vi "通信模块_串口调试工具.vi"() -> ()   [LabVIEW 2015]
uses:
  <vilib>/Instr/_visa.llb/VISA Find Search Mode.ctl
  <vilib>/event_ctls.llb/eventvkey.ctl
  <vilib>/Instr/_visa.llb/VISA Configure Serial Port (Instr).vi
panel:
  in  "1A":bool caption="进制"
  in  "2 3":string
  in  "2 2":bool
  in  "1 3":string
  in  "1 2":bool
  in  "5 3":bool
  in  "4 3":bool
  in  "3 3":bool
  in  "5 2":string
  in  "4 2":string
  in  "3 2":string
  in  "ATI":bool
  in  "CGMM":bool
  in  "CGMI":bool
  in  "ATE1":bool
  in  "批量AT":bool
  in  "保存":bool
  in  "时间显示":bool caption="进制"
  in  "CGMR":bool
  in  "回车":bool=TRUE caption="进制"
  in  "十六进制":bool caption="进制"
  in  "2":string
  in  "2":bool
  in  "1":string
  in  "1":bool
  in  "语音":bool
  in  "短信":bool
  in  "ATE0":bool
  in  "CIMI":bool
  in  "CREG":bool
  in  "CPIN?":bool
  in  "CSQ":bool
  in  "5":bool
  in  "4":bool
  in  "3":bool
  in  "AT+？ 5":bool
  in  "5":string
  in  "4":string
  in  "3":string
  in  "AT+? 5":string
  in  "手动发送":bool
  in  "周期":u16=100
  in  "自动发送":bool
  in  "发送区":string
  in  "AT+? 4":bool
  in  "AT+? 4":string
  out "发送":string
  in  "窗口":string
  in  "AT+？ 3":bool
  in  "AT+? 3":string
  in  "AT+？ 2":bool
  in  "AT+? 2":string
  in  "AT+？":bool
  in  "AT+? 1":string
  in  "AT":bool
  in  "清空":bool
  out "VISA":refnum<visa-resource-name>
  in  "端口":string(combo)="COM2"
  in  "波特率":string(combo)="115200"
  out "布尔":bool
  in  "串口开关":bool
  # "毫秒"
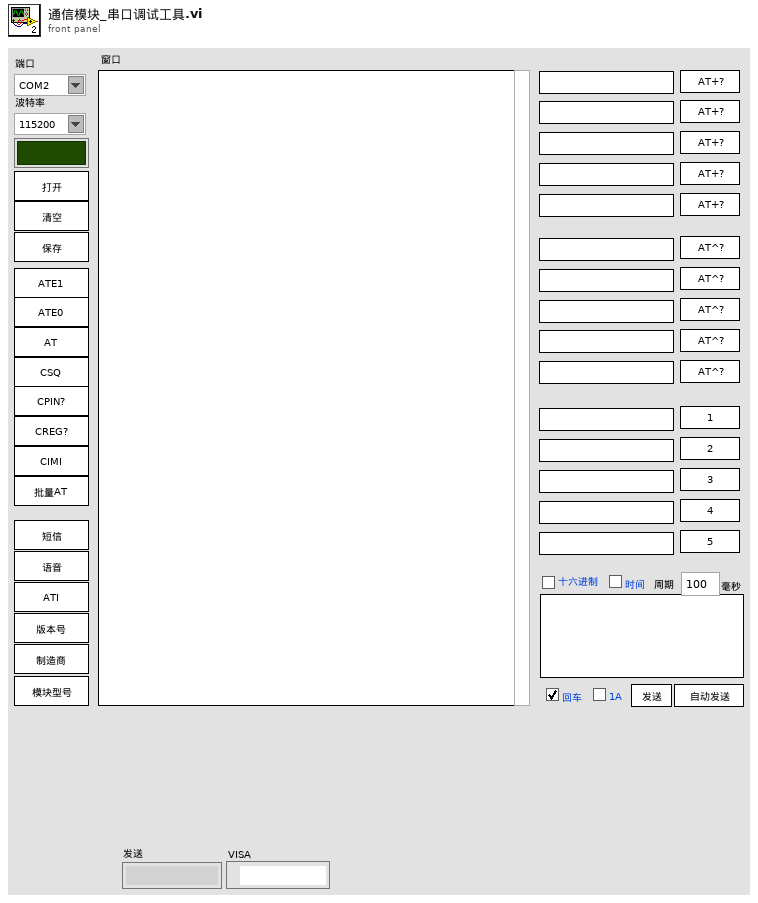
[diagram p1: front panel]
types:
  T1 = typedef "VISA Find Search Mode.ctl" = u32
  T2 = typedef "eventvkey.ctl" = enum16{"ASCII", "Enter", "Return", "Shift", "Ctrl", "Alt", "Cmd", "Opt", "Caps", "NumLock", "Clear", "Break", "Up", "Down", "Left", "Right", "Insert", "Delete", "Home", "End", "PageUp", "PageDown", "Escape", "Help", "Pause", "ScrollLock", "F1", "F2", "F3", "F4", "F5", "F6", "F7", "F8", "F9", "F10", "F11", "F12", "F13", "F14", "F15", "F16", "F17", "F18", "F19", "F20", "F21", "F22", "F23", "F24", "Play", "VolumeUp", "VolumeDown", "Mute", "Two Byte Char"}
  T3 = cluster{"Shift":bool, "Ctrl":bool, "Alt":bool, "Cmd":bool, "Opt":bool}
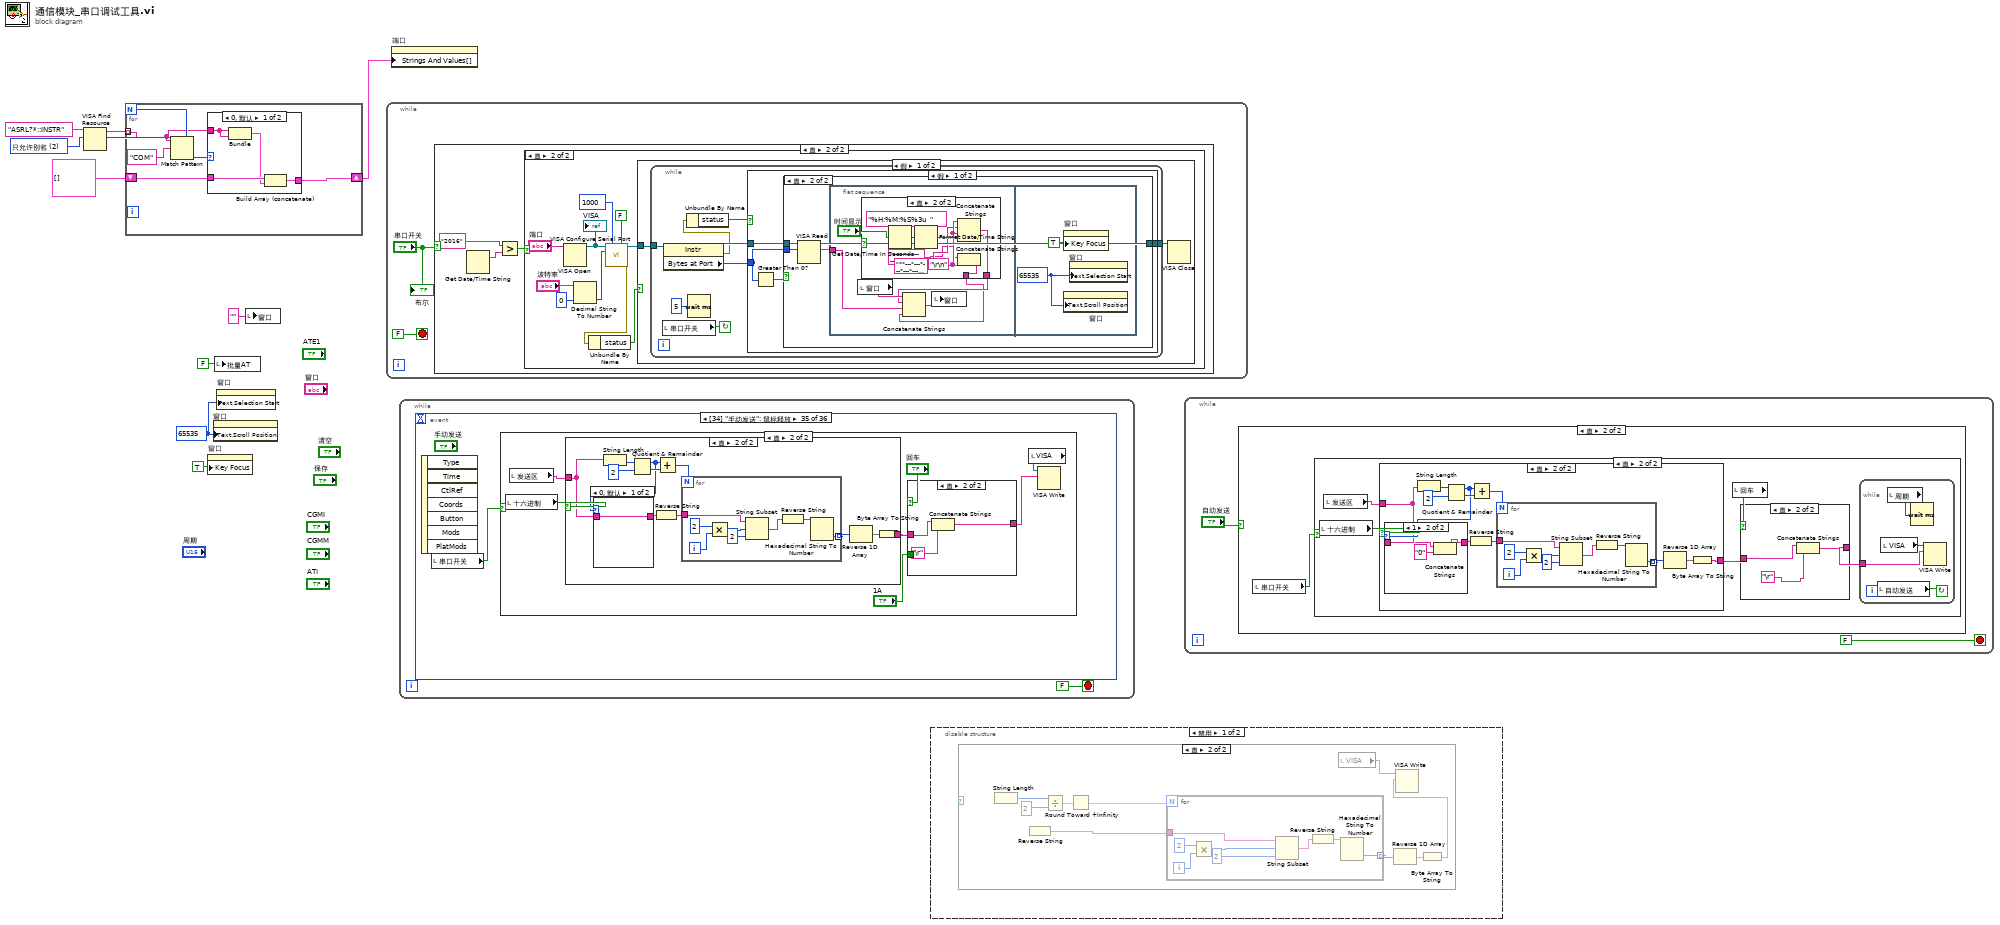
[diagram p0: block diagram]
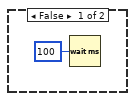
[diagram p3: hidden frame]
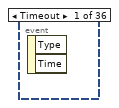
[diagram p10: hidden frame]
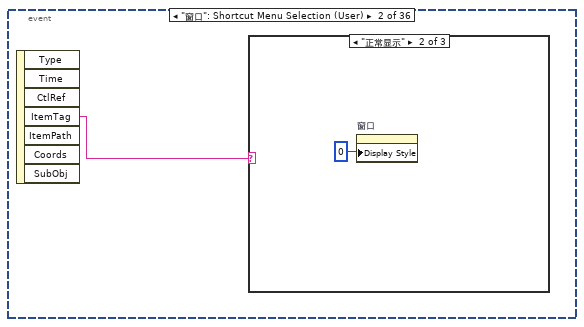
[diagram p11: hidden frame]
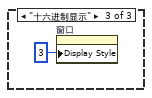
[diagram p13: hidden frame]
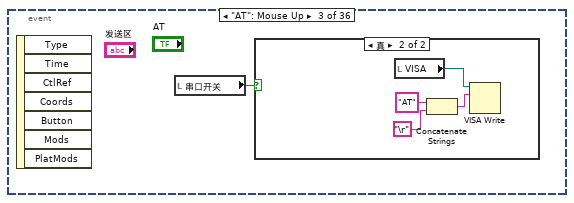
[diagram p14: hidden frame]
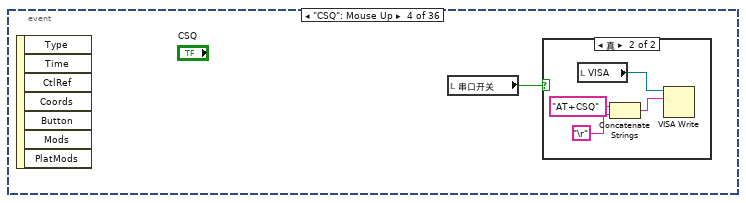
[diagram p16: hidden frame]
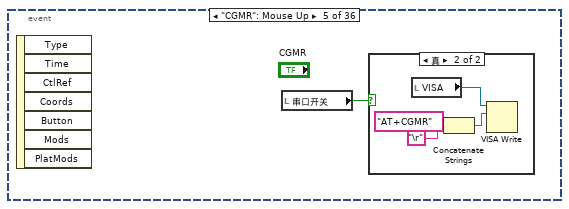
[diagram p18: hidden frame]
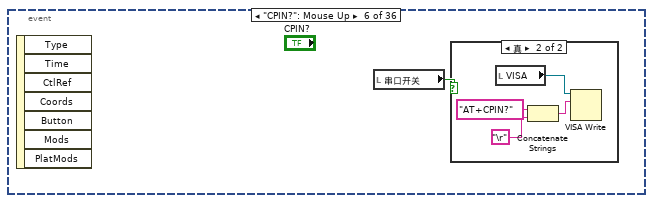
[diagram p20: hidden frame]
diagram:
  w3 = T1 2 items=["仅允许规范名称"=0, "只允许别名"=2, "包含匹配别名"=3, "包含所有别名"=4] ("Search Mode")
  w9 = u32 65535 ("文本.滚动条位置")
  n1 = VISA Find Resource(10:w3, 11:"ASRL?*::INSTR") -> (2:w7:u32, 3:w6:string[])  [unwired: 1 in, 1 out]
  n2 = for {
    N: w7 -> [_]
    tunnel: w6 -> [w13] mode=indexing
    shift-right: [w12] -> w1
    shift-left: cluster{string, string}[] [] -> [w11]
    n3 = Match Pattern(string=w13, regular expression="COM" ("正则表达式")) -> (offset past match=w14:i32)  [unwired: 1 in, 3 out]
    n4 = case shown="0, 默认" w14 {
      tunnel: w11 -> [w19 w20]
      tunnel: w13 -> [w17 _]
      tunnel: [w18 w20] -> w12
      frame 0, Default {
        n5 = Bundle(w17, w17) -> (w16:cluster{string, string})  [unwired: 1 in]
        n6 = Build Array (concatenate)(w19, w16) -> (w18:cluster{string, string}[])
      }
      frame -1 {
      }
    }
  }
  n7 = property on="窗口" class="Str"("Key Focus"=TRUE ("键选中")) -> ()  [unwired: 2 in, 2 out]
  n8 = property on="窗口" class="Str"("Text.Scroll Position"=w9) -> ()  [unwired: 2 in, 2 out]
  n9 = local write "批量AT"(FALSE ("批量AT")) -> ()
  n10 = property on="窗口" class="Str"("Text.Selection Start"=w9) -> ()  [unwired: 2 in, 2 out]
  n11 = local write "窗口"("" ("窗口")) -> ()
  n12 = while {
    stop <- FALSE stop-if-true
    n13 = case shown="真" "串口开关" {
      frame False {
        n14 = Wait (ms)(milliseconds to wait=u32 100 ("等待时间（毫秒）")) -> ()  [unwired: 1 out]
      }
      frame True {
        n15 = Get Date/Time String() -> (date string=w26:string)  [unwired: 3 in, 1 out]
        n16 = Greater?(x="2016", y=w26) -> (0:w24:bool)
        n17 = case shown="真" w24 {
          frame False {
            n18 = Wait (ms)(milliseconds to wait=u32 100 ("等待时间（毫秒）")) -> ()  [unwired: 1 out]
          }
          frame True {
            n19 = VISA Open(VISA resource name="端口") -> (VISA resource name=w37:refnum<visa-resource-name>)  [unwired: 4 in, 1 out]
            "VISA" <- w37
            n20 = Decimal String To Number(string="波特率", default (0L)=u32 0 ("默认(0 I32)")) -> (number=w30:u32)  [unwired: 1 in, 1 out]
            n21 = call-poly "VISA Configure Serial Port"("VISA resource name"=w37, "timeout (10sec)"=u32 1000, "Enable Termination\nChar (T)"=FALSE ("Enable Termination\nChar (T)"), "baud rate (9600)"=w30) -> ("VISA resource name out"=w34:refnum<visa-resource-name>, "error out"=w33:errorcluster)  [unwired: 10 in]
            n22 = Unbundle By Name(w33) -> ("status"=w32:bool)
            n23 = case shown="假" w32 {
              tunnel: w34 -> [w38 _]
              frame False {
                n24 = while {
                  tunnel: [w45] -> w39
                  tunnel: w38 -> [w43]
                  stop <- w47 continue-if-true
                  n25 = local read "串口开关"() -> (w47:bool)
                  n26 = property class="Instr"(reference=w43) -> (reference out=w46:refnum<visa-resource-name>, error out=w41:errorcluster, "Bytes at Port"=w42:u32)  [unwired: 1 in]
                  n27 = Unbundle By Name(w41) -> ("status"=w40:bool)
                  n28 = Wait (ms)(milliseconds to wait=u32 5 ("等待时间（毫秒）")) -> ()  [unwired: 1 out]
                  n29 = case shown="假" w40 {
                    tunnel: w46 -> [w51 w74]
                    tunnel: [w50 w74] -> w45
                    tunnel: w42 -> [w48 _]
                    frame False {
                      n30 = Greater Than 0?(x=w48) -> (x > 0?=w49:bool)
                      n31 = case shown="真" w49 {
                        tunnel: w51 -> [w52 w56]
                        tunnel: w48 -> [_ w55]
                        tunnel: [w52 w54] -> w50
                        frame False {
                        }
                        frame True {
                          n32 = VISA Read(VISA resource name=w56, byte count=w55) -> (VISA resource name out=w54:refnum<visa-resource-name>, read buffer=w53:string)  [unwired: 1 in, 2 out]
                          n33 = flat-sequence {
                            tunnel: w53 -> [w59]
                            frame #0 {
                              n34 = local read "窗口"() -> (w61:string)
                              n35 = case shown="真" "时间显示" {
                                tunnel: [w63 w68] -> w58
                                tunnel: [w63 w66] -> w57
                                frame False {
                                w63 = "" ("date/time string")
                                }
                                frame True {
                                w67 = "\r\n"
                                n36 = Get Date/Time In Seconds() -> (seconds since 1Jan1904=w71:timestamp)
                                n37 = Format Date/Time String(time format string (%c)="%H:%M:%S%3u  " ("时间格式字符串(%c)"), seconds (now)=w71) -> (date/time string=w69:string)  [unwired: 1 in]
                                n38 = Concatenate Strings(w67, "**---*---*---*---*---*---*---*---*---*---*---*---*---*---*---**" ("窗口"), w67, w69) -> (w68:string)
                                n39 = Concatenate Strings("----------------------------------------------------------------" ("窗口"), w67) -> (w66:string)
                                }
                              }
                              n40 = Concatenate Strings(w61, w58, w59, w57) -> (w62:string)
                              n41 = local write "窗口"(w62) -> ()
                            }
                            frame #1 {
                              w72 = u32 65535 ("文本.选择区域:起始")
                              n42 = property on="窗口" class="Str"("Key Focus"=TRUE ("键选中")) -> ()  [unwired: 2 in, 2 out]
                              n43 = property on="窗口" class="Str"("Text.Scroll Position"=w72) -> ()  [unwired: 2 in, 2 out]
                              n44 = property on="窗口" class="Str"("Text.Selection Start"=w72) -> ()  [unwired: 2 in, 2 out]
                            }
                          }
                        }
                      }
                    }
                    frame True {
                    }
                  }
                }
                n45 = VISA Close(VISA resource name=w39) -> ()  [unwired: 1 in, 1 out]
              }
              frame True {
                n46 = flat-sequence {
                  frame #0 {
                    n47 = local read "端口"() -> (w77:string)
                    n48 = Concatenate Strings(w77, "打开失败！" ("字符串")) -> (w75:string)
                    n49 = One Button Dialog(message=w75) -> ()  [unwired: 1 in, 1 out]
                  }
                  frame #1 {
                    n50 = local write "串口开关"(FALSE ("串口开关")) -> ()
                  }
                }
              }
            }
          }
        }
      }
    }
    "布尔" <- "串口开关"
  }
  n51 = property on="端口" class="CmbBox"("Strings And Values[]"=w1) -> ()  [unwired: 2 in, 2 out]
  n52 = while {
    stop <- FALSE stop-if-true
    n53 = event shown="[34] \"手动发送\": 鼠标释放" {
      selector: _ -> [_ _ _ _ _ _ _ _ _ _ _ _ _ _ _ _ _ _ _ _ _ _ _ _ _ _ _ _ _ _ _ _ _ _ _ _]
      dyn-events: _ -> [_ _ _ _ _ _ _ _ _ _ _ _ _ _ _ _ _ _ _ _ _ _ _ _ _ _ _ _ _ _ _ _ _ _ _ _]
      timeout: _ -> [_ _ _ _ _ _ _ _ _ _ _ _ _ _ _ _ _ _ _ _ _ _ _ _ _ _ _ _ _ _ _ _ _ _ _ _]
      event Timeout {
        n54 = event-data() -> ()  [unwired: 1 in, 2 out]
      }
      event "窗口": Shortcut Menu Selection (User) {
        n55 = event-data() -> ("ItemTag"=w80:string)  [unwired: 1 in, 6 out]
        n56 = case shown="\"正常显示\"" w80 {
          frame "假", Default {
          }
          frame "正常显示" {
            n57 = property on="窗口" class="Str"("Display Style"=u32 0 ("显示样式")) -> ()  [unwired: 2 in, 2 out]
          }
          frame "十六进制显示" {
            n58 = property on="窗口" class="Str"("Display Style"=u32 3 ("显示样式")) -> ()  [unwired: 2 in, 2 out]
          }
        }
      }
      event "AT": Mouse Up {
        n59 = event-data() -> ()  [unwired: 1 in, 7 out]
        n60 = local read "串口开关"() -> (w83:bool)
        n61 = case shown="真" w83 {
          frame False {
          }
          frame True {
            n62 = local read "VISA"() -> (w87:refnum<visa-resource-name>)
            n63 = Concatenate Strings("AT" ("字符串"), "\r") -> (w86:string)
            n64 = VISA Write(VISA resource name=w87, write buffer=w86) -> ()  [unwired: 1 in, 3 out]
          }
        }
      }
      event "CSQ": Mouse Up {
        n65 = event-data() -> ()  [unwired: 1 in, 7 out]
        n66 = local read "串口开关"() -> (w88:bool)
        n67 = case shown="真" w88 {
          frame False {
          }
          frame True {
            n68 = local read "VISA"() -> (w92:refnum<visa-resource-name>)
            n69 = Concatenate Strings("AT+CSQ" ("字符串"), "\r") -> (w91:string)
            n70 = VISA Write(VISA resource name=w92, write buffer=w91) -> ()  [unwired: 1 in, 3 out]
          }
        }
      }
      event "CGMR": Mouse Up {
        n71 = event-data() -> ()  [unwired: 1 in, 7 out]
        n72 = local read "串口开关"() -> (w93:bool)
        n73 = case shown="真" w93 {
          frame False {
          }
          frame True {
            n74 = local read "VISA"() -> (w97:refnum<visa-resource-name>)
            n75 = Concatenate Strings("AT+CGMR" ("字符串"), "\r") -> (w96:string)
            n76 = VISA Write(VISA resource name=w97, write buffer=w96) -> ()  [unwired: 1 in, 3 out]
          }
        }
      }
      event "CPIN?": Mouse Up {
        n77 = event-data() -> ()  [unwired: 1 in, 7 out]
        n78 = local read "串口开关"() -> (w98:bool)
        n79 = case shown="真" w98 {
          frame False {
          }
          frame True {
            n80 = local read "VISA"() -> (w102:refnum<visa-resource-name>)
            n81 = Concatenate Strings("AT+CPIN?" ("字符串"), "\r") -> (w101:string)
            n82 = VISA Write(VISA resource name=w102, write buffer=w101) -> ()  [unwired: 1 in, 3 out]
          }
        }
      }
      event "CREG": Mouse Up {
        n83 = event-data() -> ()  [unwired: 1 in, 7 out]
        n84 = local read "串口开关"() -> (w103:bool)
        n85 = case shown="真" w103 {
          frame False {
          }
          frame True {
            n86 = local read "VISA"() -> (w107:refnum<visa-resource-name>)
            n87 = Concatenate Strings("AT+CREG?" ("字符串"), "\r") -> (w106:string)
            n88 = VISA Write(VISA resource name=w107, write buffer=w106) -> ()  [unwired: 1 in, 3 out]
          }
        }
      }
      event "CIMI": Mouse Up {
        n89 = event-data() -> ()  [unwired: 1 in, 7 out]
        n90 = local read "串口开关"() -> (w108:bool)
        n91 = case shown="真" w108 {
          frame False {
          }
          frame True {
            n92 = local read "VISA"() -> (w112:refnum<visa-resource-name>)
            n93 = Concatenate Strings("AT+CIMI" ("字符串"), "\r") -> (w111:string)
            n94 = VISA Write(VISA resource name=w112, write buffer=w111) -> ()  [unwired: 1 in, 3 out]
          }
        }
      }
      event "ATE0": Mouse Up {
        n95 = event-data() -> ()  [unwired: 1 in, 7 out]
        n96 = local read "串口开关"() -> (w113:bool)
        n97 = case shown="真" w113 {
          frame False {
          }
          frame True {
            n98 = local read "VISA"() -> (w117:refnum<visa-resource-name>)
            n99 = Concatenate Strings("ATE0" ("字符串"), "\r") -> (w116:string)
            n100 = VISA Write(VISA resource name=w117, write buffer=w116) -> ()  [unwired: 1 in, 3 out]
          }
        }
      }
      event "短信": Mouse Up {
        n101 = event-data() -> ()  [unwired: 1 in, 7 out]
        n102 = flat-sequence {
          frame #0 {
            n103 = local read "VISA"() -> (w121:refnum<visa-resource-name>)
            n104 = Concatenate Strings("AT+CMGS=13" ("字符串"), "\r") -> (w120:string)
            n105 = VISA Write(VISA resource name=w121, write buffer=w120) -> ()  [unwired: 1 in, 3 out]
          }
          frame #1 {
            n106 = Wait (ms)(milliseconds to wait=u32 1000 ("等待时间（毫秒）")) -> ()  [unwired: 1 out]
          }
          frame #2 {
            n107 = local read "VISA"() -> (w125:refnum<visa-resource-name>)
            n108 = Concatenate Strings("00110005810180F60000AA026235" ("字符串"), "\u001a" ("字符串")) -> (w126:string)
            n109 = VISA Write(VISA resource name=w125, write buffer=w126) -> ()  [unwired: 1 in, 3 out]
          }
        }
      }
      event "语音": Mouse Up {
        n110 = event-data() -> ()  [unwired: 1 in, 7 out]
        n111 = flat-sequence {
          frame #0 {
            n112 = local read "VISA"() -> (w130:refnum<visa-resource-name>)
            n113 = Concatenate Strings("ATD10086;" ("字符串"), "\r") -> (w129:string)
            n114 = VISA Write(VISA resource name=w130, write buffer=w129) -> ()  [unwired: 1 in, 3 out]
          }
          frame #1 {
            n115 = Wait (ms)(milliseconds to wait=u32 10000 ("等待时间（毫秒）")) -> ()  [unwired: 1 out]
          }
          frame #2 {
            n116 = local read "VISA"() -> (w133:refnum<visa-resource-name>)
            n117 = Concatenate Strings("ATH" ("字符串"), "\r") -> (w134:string)
            n118 = VISA Write(VISA resource name=w133, write buffer=w134) -> ()  [unwired: 1 in, 3 out]
          }
        }
      }
      event "ATI": Mouse Down {
        n119 = event-data() -> ()  [unwired: 1 in, 7 out]
        n120 = local read "串口开关"() -> (w136:bool)
        n121 = case shown="真" w136 {
          frame False {
          }
          frame True {
            n122 = local read "VISA"() -> (w140:refnum<visa-resource-name>)
            n123 = Concatenate Strings("ATI" ("字符串"), "\r") -> (w139:string)
            n124 = VISA Write(VISA resource name=w140, write buffer=w139) -> ()  [unwired: 1 in, 3 out]
          }
        }
      }
      event "CGMI": Mouse Down {
        n125 = event-data() -> ()  [unwired: 1 in, 7 out]
        n126 = local read "串口开关"() -> (w141:bool)
        n127 = case shown="真" w141 {
          frame False {
          }
          frame True {
            n128 = local read "VISA"() -> (w145:refnum<visa-resource-name>)
            n129 = Concatenate Strings("AT+CGMI" ("字符串"), "\r") -> (w144:string)
            n130 = VISA Write(VISA resource name=w145, write buffer=w144) -> ()  [unwired: 1 in, 3 out]
          }
        }
      }
      event "CGMM": Mouse Down {
        n131 = event-data() -> ()  [unwired: 1 in, 7 out]
        n132 = local read "串口开关"() -> (w146:bool)
        n133 = case shown="真" w146 {
          frame False {
          }
          frame True {
            n134 = local read "VISA"() -> (w150:refnum<visa-resource-name>)
            n135 = Concatenate Strings("AT+CGMM" ("字符串"), "\r") -> (w149:string)
            n136 = VISA Write(VISA resource name=w150, write buffer=w149) -> ()  [unwired: 1 in, 3 out]
          }
        }
      }
      event "ATE1": Mouse Up {
        n137 = event-data() -> ()  [unwired: 1 in, 7 out]
        n138 = local read "VISA"() -> (w152:refnum<visa-resource-name>)
        n139 = Concatenate Strings("ATE1" ("字符串"), "\r") -> (w153:string)
        n140 = VISA Write(VISA resource name=w152, write buffer=w153) -> ()  [unwired: 1 in, 3 out]
      }
      event "窗口": Key Down {
        n141 = event-data() -> ("Char"=w161:i16, "VKey"=w157:T2, "PlatMods"=w156:T3)  [unwired: 1 in, 6 out]
        n142 = Unbundle By Name(w156) -> ("Ctrl"=w155:bool)
        n143 = In Range and Coerce(upper limit=eventvkey."Shift" ("上限"), x=w157, lower limit=eventvkey."Enter" ("下限")) -> (In Range?=w158:bool)  [unwired: 1 out]
        n144 = case shown="真" w158 {
          tunnel: w161 -> [w163 _]
          tunnel: w155 -> [w162 _]
          frame False {
            n145 = case shown="真" w162 {
              tunnel: w163 -> [w167 w182]
              frame False {
                n146 = In Range and Coerce(upper limit=i16 126 ("上限"), x=w167, lower limit=i16 32 ("下限")) -> (In Range?=w166:bool)  [unwired: 1 out]
                n147 = case shown="假" w166 {
                  tunnel: w167 -> [w170 w176]
                  frame False {
                    n148 = Equal?(x=w170, y=i16 8) -> (x = y?=w168:bool)
                    n149 = case shown="假" w168 {
                      frame False {
                      }
                      frame True {
                        n150 = local read "发送"() -> (w172:string)
                        n151 = String Length(string=w172) -> (length=w173:i32)
                        n152 = Decrement(x=w173) -> (x-1=w174:i32)
                        n153 = String Subset(string=w172, length (rest)=w174) -> (substring=w171:string)  [unwired: 1 in]
                        n154 = local write "发送"(w171) -> ()
                      }
                    }
                  }
                  frame True {
                    n155 = Build Array(w176) -> (w177:i16[])
                    n156 = local read "发送"() -> (w179:string)
                    n157 = Byte Array To String(unsigned byte array=w177) -> (string=w175:string)
                    n158 = Concatenate Strings(w179, w175) -> (w178:string)
                    n159 = local write "发送"(w178) -> ()
                  }
                }
              }
              frame True {
                n160 = Equal?(x=w182, y=i16 97) -> (x = y?=w180:bool)
                n161 = case shown="真" w180 {
                  frame False {
                  }
                  frame True {
                    n162 = flat-sequence {
                      tunnel: [w188] -> w186
                      tunnel: [w187] -> w184
                      frame #0 {
                        n163 = local read "窗口"() -> (w188:string)
                        n164 = String Length(string=w188) -> (length=w187:i32)
                        n165 = property on="窗口" class="Str"("Key Focus"=TRUE ("键选中"), "Text.Selection Start"=u32 0 ("文本.选择区域:起始"), "Text.Selection End"=w187) -> ()  [unwired: 2 in, 2 out]
                      }
                    }
                    n166 = Decrement(x=w184) -> (x-1=w185:i32)
                    n167 = String Subset(string=w186, length (rest)=w185) -> (substring=w183:string)  [unwired: 1 in]
                    n168 = local write "窗口"(w183) -> ()
                  }
                }
              }
            }
          }
          frame True {
            n169 = stacked-sequence {
              frame #0 {
                n170 = local read "发送"() -> (w192:string)
                n171 = local read "VISA"() -> (w194:refnum<visa-resource-name>)
                n172 = Concatenate Strings(w192, "\r") -> (w193:string)
                n173 = VISA Write(VISA resource name=w194, write buffer=w193) -> ()  [unwired: 1 in, 3 out]
              }
              frame #1 {
                n174 = local write "发送"("" ("发送")) -> ()
              }
            }
          }
        }
      }
      event "清空": Mouse Up {
        n175 = event-data() -> ()  [unwired: 1 in, 7 out]
        n176 = local write "窗口"("") -> ()
        n177 = property on="窗口" class="Str"("Key Focus"=TRUE ("键选中")) -> ()  [unwired: 2 in, 2 out]
      }
      event "AT+？": Mouse Up {
        n178 = event-data() -> ()  [unwired: 1 in, 7 out]
        n179 = local read "串口开关"() -> (w198:bool)
        n180 = case shown="真" w198 {
          frame False {
          }
          frame True {
            n181 = local read "VISA"() -> (w203:refnum<visa-resource-name>)
            n182 = Concatenate Strings("AT+" ("字符串"), "AT+? 1", "\r") -> (w202:string)
            n183 = VISA Write(VISA resource name=w203, write buffer=w202) -> ()  [unwired: 1 in, 3 out]
          }
        }
      }
      event "AT+？ 2": Mouse Up {
        n184 = event-data() -> ()  [unwired: 1 in, 7 out]
        n185 = local read "串口开关"() -> (w204:bool)
        n186 = case shown="真" w204 {
          frame False {
          }
          frame True {
            n187 = local read "VISA"() -> (w209:refnum<visa-resource-name>)
            n188 = Concatenate Strings("AT+" ("字符串"), "AT+? 2", "\r") -> (w208:string)
            n189 = VISA Write(VISA resource name=w209, write buffer=w208) -> ()  [unwired: 1 in, 3 out]
          }
        }
      }
      event "AT+？ 3": Mouse Up {
        n190 = event-data() -> ()  [unwired: 1 in, 7 out]
        n191 = local read "串口开关"() -> (w210:bool)
        n192 = case shown="真" w210 {
          frame False {
          }
          frame True {
            n193 = local read "VISA"() -> (w215:refnum<visa-resource-name>)
            n194 = Concatenate Strings("AT+" ("字符串"), "AT+? 3", "\r") -> (w214:string)
            n195 = VISA Write(VISA resource name=w215, write buffer=w214) -> ()  [unwired: 1 in, 3 out]
          }
        }
      }
      event "AT+? 4": Mouse Up {
        n196 = event-data() -> ()  [unwired: 1 in, 7 out]
        n197 = local read "串口开关"() -> (w216:bool)
        n198 = case shown="真" w216 {
          frame False {
          }
          frame True {
            n199 = local read "VISA"() -> (w221:refnum<visa-resource-name>)
            n200 = Concatenate Strings("AT+" ("字符串"), "AT+? 4", "\r") -> (w220:string)
            n201 = VISA Write(VISA resource name=w221, write buffer=w220) -> ()  [unwired: 1 in, 3 out]
          }
        }
      }
      event "AT+？ 5": Mouse Up {
        n202 = event-data() -> ()  [unwired: 1 in, 7 out]
        n203 = local read "串口开关"() -> (w222:bool)
        n204 = case shown="真" w222 {
          frame False {
          }
          frame True {
            n205 = local read "VISA"() -> (w227:refnum<visa-resource-name>)
            n206 = Concatenate Strings("AT+" ("字符串"), "AT+? 5", "\r") -> (w226:string)
            n207 = VISA Write(VISA resource name=w227, write buffer=w226) -> ()  [unwired: 1 in, 3 out]
          }
        }
      }
      event "1 2": Mouse Down {
        n208 = event-data() -> ()  [unwired: 1 in, 7 out]
        n209 = local read "串口开关"() -> (w228:bool)
        n210 = case shown="真" w228 {
          frame False {
          }
          frame True {
            n211 = local read "VISA"() -> (w233:refnum<visa-resource-name>)
            n212 = Concatenate Strings("AT^" ("字符串"), "1 3", "\r") -> (w232:string)
            n213 = VISA Write(VISA resource name=w233, write buffer=w232) -> ()  [unwired: 1 in, 3 out]
          }
        }
      }
      event "2 2": Mouse Down {
        n214 = event-data() -> ()  [unwired: 1 in, 7 out]
        n215 = local read "串口开关"() -> (w234:bool)
        n216 = case shown="真" w234 {
          frame False {
          }
          frame True {
            n217 = local read "VISA"() -> (w239:refnum<visa-resource-name>)
            n218 = Concatenate Strings("AT^" ("字符串"), "2 3", "\r") -> (w238:string)
            n219 = VISA Write(VISA resource name=w239, write buffer=w238) -> ()  [unwired: 1 in, 3 out]
          }
        }
      }
      event "3 3": Mouse Down {
        n220 = event-data() -> ()  [unwired: 1 in, 7 out]
        n221 = local read "串口开关"() -> (w240:bool)
        n222 = case shown="真" w240 {
          frame False {
          }
          frame True {
            n223 = local read "VISA"() -> (w245:refnum<visa-resource-name>)
            n224 = Concatenate Strings("AT^" ("字符串"), "3 2", "\r") -> (w244:string)
            n225 = VISA Write(VISA resource name=w245, write buffer=w244) -> ()  [unwired: 1 in, 3 out]
          }
        }
      }
      event "4 3": Mouse Down {
        n226 = event-data() -> ()  [unwired: 1 in, 7 out]
        n227 = local read "串口开关"() -> (w246:bool)
        n228 = case shown="真" w246 {
          frame False {
          }
          frame True {
            n229 = local read "VISA"() -> (w251:refnum<visa-resource-name>)
            n230 = Concatenate Strings("AT^" ("字符串"), "4 2", "\r") -> (w250:string)
            n231 = VISA Write(VISA resource name=w251, write buffer=w250) -> ()  [unwired: 1 in, 3 out]
          }
        }
      }
      event "5 3": Mouse Down {
        n232 = event-data() -> ()  [unwired: 1 in, 7 out]
        n233 = local read "串口开关"() -> (w252:bool)
        n234 = case shown="真" w252 {
          frame False {
          }
          frame True {
            n235 = local read "VISA"() -> (w257:refnum<visa-resource-name>)
            n236 = Concatenate Strings("AT^" ("字符串"), "5 2", "\r") -> (w256:string)
            n237 = VISA Write(VISA resource name=w257, write buffer=w256) -> ()  [unwired: 1 in, 3 out]
          }
        }
      }
      event "3": Mouse Up {
        n238 = event-data() -> ()  [unwired: 1 in, 7 out]
        n239 = local read "串口开关"() -> (w258:bool)
        n240 = case shown="真" w258 {
          frame False {
          }
          frame True {
            n241 = local read "VISA"() -> (w262:refnum<visa-resource-name>)
            n242 = Concatenate Strings("3", "\r") -> (w261:string)
            n243 = VISA Write(VISA resource name=w262, write buffer=w261) -> ()  [unwired: 1 in, 3 out]
          }
        }
      }
      event "保存": Mouse Up {
        w272 = "" ("替换字符串(\"\")")
        n244 = event-data() -> ()  [unwired: 1 in, 7 out]
        n245 = Get Date/Time String() -> (date string=w276:string, time string=w274:string)  [unwired: 3 in]
        n246 = Search and Replace String(replace all?=TRUE ("替换全部？(F)"), input string=w276, search string="-" ("搜索字符串"), replace string=w272) -> (result string=w269:string)  [unwired: 4 in, 3 out]
        n247 = Search and Replace String(input string=w274, search string=":" ("搜索字符串"), replace string=w272) -> (result string=w270:string)  [unwired: 5 in, 3 out]
        n248 = Concatenate Strings("乐卡调试内容" ("字符串"), w269, w270) -> (w268:string)
        n249 = call "文件对话框"("start path"=path "D:/", "prompt"="内容保存", "button label"="保存", "default name"=w268, "pattern (all files)"="*.txt", "pattern label"="文本文件") -> ("selected path"=w280:path, "cancelled"=w264:bool, "error out"=w279:errorcluster)  [unwired: 6 in, 1 out]
        n250 = case shown="假" w264 {
          tunnel: w280 -> [w283 _]
          tunnel: w279 -> [w282 _]
          frame False {
            n251 = local read "窗口"() -> (w284:string)
            n252 = Write to Text File(file (use dialog)=w283, text=w284, error in=w282) -> (error out=w281:errorcluster)  [unwired: 1 in, 2 out]
            n253 = call <vilib>:"Clear Errors.vi"("error in (no error)"=w281) -> ()  [unwired: 5 in, 2 out]
          }
          frame True {
          }
        }
      }
      event "批量AT": Value Change {
        n254 = event-data() -> ()  [unwired: 1 in, 5 out]
        n255 = local read "串口开关"() -> (w285:bool)
        n256 = case shown="真" w285 {
          frame False {
            n257 = local write "批量AT"(FALSE ("批量AT")) -> ()
          }
          frame True {
            n258 = stacked-sequence {
              frame #0 {
                n259 = local read "批量AT"() -> (w287:bool)
                n260 = case shown="真" w287 {
                  frame False {
                  }
                  frame True {
                    n261 = call "文件对话框2"("start path"=path "D:/") -> ("selected path"=w289:path, "exists"=w290:bool)  [unwired: 11 in, 2 out]
                    n262 = case shown="真" w290 {
                      tunnel: w289 -> [_ w292]
                      frame False {
                      }
                      frame True {
                        n263 = Read from Text File(file (use dialog)=w292) -> (text=w291:string)  [unwired: 3 in, 3 out]
                        n264 = while {
                          shift-right: [w313] -> _
                          shift-left: w291 -> [w312]
                          stop <- w315 continue-if-true
                          n265 = Match Pattern(string=w312, regular expression="[\\n\\r]+" ("正则表达式")) -> (before substring=w311:string, after substring=w313:string, offset past match=w314:i32)  [unwired: 1 in, 1 out]
                          n266 = Greater Than 0?(x=w314) -> (x > 0?=w317:bool)
                          n267 = And(x=w317, y="批量AT") -> (x .and. y?=w315:bool)
                          n268 = Match Pattern(string=w311, regular expression="[/\\][/\\]" ("正则表达式")) -> (before substring=w301:string, after substring=w308:string)  [unwired: 1 in, 2 out]
                          n269 = Match Pattern(string=w308, regular expression="@" ("正则表达式")) -> (before substring=w298:string, after substring=w306:string)  [unwired: 1 in, 2 out]
                          n270 = Match Pattern(string=w301, regular expression="[\\t]+" ("正则表达式")) -> (before substring=w300:string)  [unwired: 1 in, 3 out]
                          n271 = Match Pattern(string=w298, regular expression="%" ("正则表达式")) -> (after substring=w294:string, offset past match=w297:i32)  [unwired: 1 in, 2 out]
                          n272 = Match Pattern(string=w306, regular expression="[0-9]+" ("正则表达式")) -> (match substring=w302:string, offset past match=w305:i32)  [unwired: 1 in, 2 out]
                          n273 = local read "VISA"() -> (w319:refnum<visa-resource-name>)
                          n274 = Greater Or Equal To 0?(x=w297) -> (x >= 0?=w296:bool)
                          n275 = Greater Or Equal To 0?(x=w305) -> (x >= 0?=w304:bool)
                          n276 = Concatenate Strings(w300, "\r") -> (w318:string)
                          n277 = case shown="真" w296 {
                            tunnel: w294 -> [_ w323]
                            frame False {
                            }
                            frame True {
                              w321 = "\r\n"
                              n278 = local read "窗口"() -> (w322:string)
                              n279 = Concatenate Strings(w322, w321, w323, w321) -> (w324:string)
                              n280 = local write "窗口"(w324) -> ()
                            }
                          }
                          n281 = case shown="真" w304 {
                            tunnel: [u32 1000 ("等待时间（毫秒）") w327] -> w303
                            tunnel: w302 -> [_ w326]
                            frame False {
                            }
                            frame True {
                              n282 = Decimal String To Number(string=w326) -> (number=w327:i32)  [unwired: 2 in, 1 out]
                            }
                          }
                          n283 = VISA Write(VISA resource name=w319, write buffer=w318) -> ()  [unwired: 1 in, 3 out]
                          n284 = Wait (ms)(milliseconds to wait=w303) -> ()  [unwired: 1 out]
                        }
                      }
                    }
                  }
                }
              }
              frame #1 {
                n285 = local write "批量AT"(FALSE ("批量AT")) -> ()
              }
            }
          }
        }
      }
      event "4": Mouse Up {
        n286 = event-data() -> ()  [unwired: 1 in, 7 out]
        n287 = local read "串口开关"() -> (w329:bool)
        n288 = case shown="真" w329 {
          frame False {
          }
          frame True {
            n289 = local read "VISA"() -> (w333:refnum<visa-resource-name>)
            n290 = Concatenate Strings("4", "\r") -> (w332:string)
            n291 = VISA Write(VISA resource name=w333, write buffer=w332) -> ()  [unwired: 1 in, 3 out]
          }
        }
      }
      event "5": Mouse Up {
        n292 = event-data() -> ()  [unwired: 1 in, 7 out]
        n293 = local read "串口开关"() -> (w334:bool)
        n294 = case shown="真" w334 {
          frame False {
          }
          frame True {
            n295 = local read "VISA"() -> (w338:refnum<visa-resource-name>)
            n296 = Concatenate Strings("5", "\r") -> (w337:string)
            n297 = VISA Write(VISA resource name=w338, write buffer=w337) -> ()  [unwired: 1 in, 3 out]
          }
        }
      }
      event "2": Mouse Up {
        n298 = event-data() -> ()  [unwired: 1 in, 7 out]
        n299 = local read "串口开关"() -> (w339:bool)
        n300 = case shown="真" w339 {
          frame False {
          }
          frame True {
            n301 = local read "VISA"() -> (w343:refnum<visa-resource-name>)
            n302 = Concatenate Strings("2", "\r") -> (w342:string)
            n303 = VISA Write(VISA resource name=w343, write buffer=w342) -> ()  [unwired: 1 in, 3 out]
          }
        }
      }
      event "1": Mouse Up {
        n304 = event-data() -> ()  [unwired: 1 in, 7 out]
        n305 = local read "串口开关"() -> (w344:bool)
        n306 = case shown="真" w344 {
          frame False {
          }
          frame True {
            n307 = local read "VISA"() -> (w348:refnum<visa-resource-name>)
            n308 = Concatenate Strings("1", "\r") -> (w347:string)
            n309 = VISA Write(VISA resource name=w348, write buffer=w347) -> ()  [unwired: 1 in, 3 out]
          }
        }
      }
      event "手动发送": Mouse Up {
        n310 = event-data() -> ()  [unwired: 1 in, 7 out]
        n311 = local read "串口开关"() -> (w349:bool)
        n312 = case shown="真" w349 {
          frame False {
          }
          frame True {
            n313 = local read "十六进制"() -> (w356:bool)
            n314 = local read "发送区"() -> (w355:string)
            n315 = case shown="真" w356 {
              tunnel: w355 -> [w367 w370]
              tunnel: [w367 w374] -> w352
              frame False {
              }
              frame True {
                n316 = String Length(string=w370) -> (length=w377:i32)
                n317 = Quotient & Remainder(x=w377, y=2) -> (x-y*floor(x/y)=w371:i32, floor(x/y)=w372:i32)
                n318 = case shown="0, 默认" w371 {
                  tunnel: w370 -> [w379 w381]
                  tunnel: [w379 w382] -> w369
                  frame 0, Default {
                  }
                  frame 1 {
                    n319 = Concatenate Strings(w381, "0" ("字符串")) -> (w382:string)
                  }
                }
                n320 = Reverse String(1:w369) -> (0:w368:string)
                n321 = Add(x=w371, y=w372) -> (x+y=w373:i32)
                n322 = for {
                  N: w373 -> [_]
                  tunnel: w368 -> [w386]
                  tunnel: [w385] -> w375 mode=indexing
                  i -> [w390]
                  n323 = Multiply(x=2, y=w390) -> (x*y=w388:i32)
                  n324 = String Subset(string=w386, offset (0)=w388, length (rest)=2 ("长度（剩余）")) -> (substring=w384:string)
                  n325 = Reverse String(1:w384) -> (0:w383:string)
                  n326 = Hexadecimal String To Number(string=w383) -> (number=w385:u32)  [unwired: 2 in, 1 out]
                }
                n327 = Reverse 1D Array(array=w375) -> (reversed array=w376:u32[])
                n328 = Byte Array To String(unsigned byte array=w376) -> (string=w374:string)
              }
            }
            n329 = case shown="真" "回车" {
              tunnel: w352 -> [w358 w365]
              tunnel: [w357 w366] -> w351
              tunnel: "1A" -> [w359 _]
              frame False {
                n330 = case shown="真" w359 {
                  tunnel: w358 -> [w360 w363]
                  tunnel: [w360 w362] -> w357
                  frame False {
                  }
                  frame True {
                    n331 = Concatenate Strings(w363, "\u001a" ("字符串")) -> (w362:string)
                  }
                }
              }
              frame True {
                n332 = Concatenate Strings(w365, "\r") -> (w366:string)
              }
            }
            n333 = local read "VISA"() -> (w354:refnum<visa-resource-name>)
            n334 = VISA Write(VISA resource name=w354, write buffer=w351) -> ()  [unwired: 1 in, 3 out]
          }
        }
      }
      event "十六进制": Value Change {
        n335 = event-data() -> ()  [unwired: 1 in, 5 out]
        n336 = disable-structure shown="禁用" {
          frame Disabled {
            n337 = case shown="假" "十六进制" {
              frame False {
                n338 = property on="发送区" class="Str"("Display Style"=u32 0 ("显示样式")) -> ()  [unwired: 2 in, 2 out]
              }
              frame True {
                n339 = property on="发送区" class="Str"("Display Style"=u32 3 ("显示样式")) -> ()  [unwired: 2 in, 2 out]
              }
            }
          }
          frame Enabled {
          }
        }
      }
    }
  }
  n340 = disable-structure shown="禁用" {
    frame Disabled {
      n341 = case shown="真" {
        selector: _ -> [_ _]
        frame False {
        }
        frame True {
          n342 = String Length() -> (length=w398:i32)  [unwired: 1 in]
          n343 = Reverse String() -> (0:w401:string)  [unwired: 1 in]
          n344 = Divide(x=w398, y=2) -> (x/y=w396:dbl)
          n345 = Round Toward +Infinity(x=w396) -> (ceil(x): smallest int >= x=w395:dbl)
          n346 = for {
            N: w395 -> [_]
            tunnel: w401 -> [w406]
            tunnel: [w405] -> w400 mode=indexing
            i -> [w410]
            n347 = Multiply(x=2, y=w410) -> (x*y=w408:i32)
            n348 = String Subset(string=w406, offset (0)=w408, length (rest)=2 ("长度（剩余）")) -> (substring=w404:string)
            n349 = Reverse String(1:w404) -> (0:w403:string)
            n350 = Hexadecimal String To Number(string=w403) -> (number=w405:u32)  [unwired: 2 in, 1 out]
          }
          n351 = local read "VISA"() -> (w402:refnum<visa-resource-name>)
          n352 = Reverse 1D Array(array=w400) -> (reversed array=w399:u32[])
          n353 = Byte Array To String(unsigned byte array=w399) -> (string=w394:string)
          n354 = VISA Write(VISA resource name=w402, write buffer=w394) -> ()  [unwired: 1 in, 3 out]
        }
      }
    }
    frame Enabled {
    }
  }
  n355 = while {
    stop <- FALSE stop-if-true
    n356 = case shown="真" "自动发送" {
      frame False {
        n357 = Wait (ms)(milliseconds to wait=u32 100 ("等待时间（毫秒）")) -> ()  [unwired: 1 out]
      }
      frame True {
        n358 = local read "串口开关"() -> (w414:bool)
        n359 = case shown="真" w414 {
          frame False {
          }
          frame True {
            n360 = local read "十六进制"() -> (w419:bool)
            n361 = local read "发送区"() -> (w418:string)
            n362 = case shown="真" w419 {
              tunnel: w418 -> [w428 w431]
              tunnel: [w428 w435] -> w417
              frame False {
              }
              frame True {
                n363 = String Length(string=w431) -> (length=w438:i32)
                n364 = Quotient & Remainder(x=w438, y=2) -> (x-y*floor(x/y)=w432:i32, floor(x/y)=w433:i32)
                n365 = case shown="1" w432 {
                  tunnel: w431 -> [w440 w442]
                  tunnel: [w440 w443] -> w430
                  frame 0, Default {
                  }
                  frame 1 {
                    n366 = Concatenate Strings(w442, "0" ("字符串")) -> (w443:string)
                  }
                }
                n367 = Reverse String(1:w430) -> (0:w429:string)
                n368 = Add(x=w432, y=w433) -> (x+y=w434:i32)
                n369 = for {
                  N: w434 -> [_]
                  tunnel: w429 -> [w447]
                  tunnel: [w446] -> w436 mode=indexing
                  i -> [w451]
                  n370 = Multiply(x=2, y=w451) -> (x*y=w449:i32)
                  n371 = String Subset(string=w447, offset (0)=w449, length (rest)=2 ("长度（剩余）")) -> (substring=w445:string)
                  n372 = Reverse String(1:w445) -> (0:w444:string)
                  n373 = Hexadecimal String To Number(string=w444) -> (number=w446:u32)  [unwired: 2 in, 1 out]
                }
                n374 = Reverse 1D Array(array=w436) -> (reversed array=w437:u32[])
                n375 = Byte Array To String(unsigned byte array=w437) -> (string=w435:string)
              }
            }
            n376 = local read "回车"() -> (w415:bool)
            n377 = case shown="真" w415 {
              tunnel: w417 -> [w420 w422]
              tunnel: [w420 w423] -> w416
              frame False {
              }
              frame True {
                n378 = Concatenate Strings(w422, "\r") -> (w423:string)
              }
            }
            n379 = while {
              tunnel: w416 -> [w424]
              stop <- w427 continue-if-true
              n380 = local read "自动发送"() -> (w427:bool)
              n381 = local read "VISA"() -> (w426:refnum<visa-resource-name>)
              n382 = local read "周期"() -> (w425:u16)
              n383 = Wait (ms)(milliseconds to wait=w425) -> ()  [unwired: 1 out]
              n384 = VISA Write(VISA resource name=w426, write buffer=w424) -> ()  [unwired: 1 in, 3 out]
            }
          }
        }
      }
    }
  }
